vi "UHR-Fleezers Control (host) - Lorentz v3.vi"() -> ()   [LabVIEW 2014] (continued)
            n2949 = call "Volt to I16.vi"("Voltage In"=w5137) -> ("I16 Voltage Out"=w5147:i16)
            n2950 = xnode "Read/Write Control"("FPGA VI Reference In"=w5153, "error in"=w5152, "AI to FIFO"=w5149, "APD to FIFO"=w5149, "Start scan (MCL)"=w5149, "AO1"=w5148, "AO2"=w5147) -> ("FPGA VI Reference Out"=w5151:T36, "error out"=w5150:errorcluster)
          }
        }
        "Initial Y" <- w5118
        "Initial X" <- w5117
        "wait to reset values" <- w5119
      }
    }
    n2951 = xnode "Read/Write Control"("FPGA VI Reference In"=w4264) -> ("FPGA VI Reference Out"=w4223:T36, "BD1 Frequency Out 1"=w4266:u64)  [unwired: 1 in, 1 out]
    n2952 = And(x="Save scans", y=w4525) -> (x .and. y?=w4545:bool)
    n2953 = call "IR AOM word to freq.vi"("Frequency Word In (U64)"=w4266) -> ("Frequency Out (MHz)"=w4265:dbl)
    n2954 = local read "BD 1 Frequency 2 (MHz)"() -> (w4325:dbl)
    n2955 = Subtract(x=w4325, y=w4265) -> (x-y=w4318:dbl)
    "Current deltaF (MHz)" <- w4318
    n2956 = control-ref of="Piezo trap cursor control"() -> (w4224:refnum<vi>)
    n2957 = Unbundle By Name("Cursor control") -> ("X"=w4226:bool, "Y"=w4225:bool)
    n2958 = local read "APD Elements/DMA read"() -> (w4382:u32)
    n2959 = local read "Trap AI Elements/DMA read"() -> (w4512:u32)
    n2960 = case shown="False" w4226 {
      tunnel: w4224 -> [w4598 w4608]
      tunnel: w4223 -> [_ w4600]
      frame False {
        n2961 = local read "T3 X (V)"() -> (w4599:dbl)
        n2962 = property class="XYGraph (strict)"(reference=w4598, "Cursor.Cursor X"=w4599) -> ()  [unwired: 1 in, 2 out]
      }
      frame True {
        n2963 = property class="XYGraph (strict)"(reference=w4608) -> ("Cursor.Cursor X"=w4605:dbl)  [unwired: 1 in, 2 out]
        n2964 = In Range and Coerce(upper limit=10.0, x=w4605, lower limit=0.0) -> (coerced(x)=w4603:dbl)  [unwired: 1 out]
        n2965 = Multiply(x=3276.7, y=w4603) -> (x*y=w4602:dbl)
        n2966 = To Unsigned Word Integer(number=w4602) -> (unsigned 16bit integer=w4601:u16)
        n2967 = xnode "Read/Write Control"("FPGA VI Reference In"=w4600, "Piezo Trap X (AO5)"=w4601) -> ()  [unwired: 1 in, 2 out]
      }
    }
    n2968 = case shown="False" w4225 {
      tunnel: w4224 -> [w4585 w4597]
      tunnel: w4223 -> [_ w4588]
      frame False {
        n2969 = local read "T3 Y (V)"() -> (w4587:dbl)
        n2970 = Negate(x=w4587) -> (-x=w4586:dbl)
        n2971 = property class="XYGraph (strict)"(reference=w4585, "Cursor.Cursor Y"=w4586) -> ()  [unwired: 1 in, 2 out]
      }
      frame True {
        n2972 = property class="XYGraph (strict)"(reference=w4597) -> ("Cursor.Cursor Y"=w4594:dbl)  [unwired: 1 in, 2 out]
        n2973 = In Range and Coerce(upper limit=0.0, x=w4594, lower limit=-10.0) -> (coerced(x)=w4593:dbl)  [unwired: 1 out]
        n2974 = Negate(x=w4593) -> (-x=w4591:dbl)
        n2975 = Multiply(x=3276.7, y=w4591) -> (x*y=w4590:dbl)
        n2976 = To Unsigned Word Integer(number=w4590) -> (unsigned 16bit integer=w4589:u16)
        n2977 = xnode "Read/Write Control"("FPGA VI Reference In"=w4588, "Piezo Trap Y (AO4)"=w4589) -> ()  [unwired: 1 in, 2 out]
      }
    }
    n2978 = local read "Trap Pos Elements/DMA read"() -> (w4473:u32)
    n2979 = local read "DMA Update Period (s)"() -> (w4300:dbl)
    n2980 = xnode "Invoke Method"("FPGA VI Reference In"=w4477, "error in"=w4476, "Number of Elements"=w4473, "Timeout (ms)"=-1) -> ("Data"=w4445:void[], "Elements Remaining"=→"Trap Pos FIFO El Remaining")  [unwired: 2 out]
    n2981 = xnode "Get Trap Data"("FPGA VI Reference In"=w4477, "error in"=w4476, "Number of Elements"=w4512, "Timeout (ms)"=-1 ("Timeout")) -> ("FPGA VI Reference Out"=w4324:T36, "error out"=w4415:errorcluster, "Data"=w4307:void[], "Elements Remaining"=w4579)
    "FIFO El. Rem." <- w4579
    n2982 = local read "Trap AI FIFO Depth"() -> (w4581:u32)
    n2983 = xnode "Get APD Data"("FPGA VI Reference In"=w4477, "error in"=w4476, "Number of Elements"=w4382, "Timeout (ms)"=-1) -> ("Data"=w4279:void[], "Elements Remaining"=→"APD FIFO Elements Remaining")  [unwired: 2 out]
    n2984 = feedback #1(0.0) -> (w4468:dbl)
    n2985 = To Time Stamp(1:w4468) -> (0:w4262:timestamp)
    n2986 = Add(x=w4300, y=w4468) -> (x+y=w4556:dbl)
    n2987 = feedback-in #1(w4556) -> ()
    n2988 = Subtract(x=w4581, y=w4512) -> (x-y=w4580:u32)
    n2989 = local read "APD Integration Time (s)"() -> (w4271:dbl)
    n2990 = Divide(x=w4579, y=w4580) -> (x/y=w4578:dbl)
    "Buffer Status" <- w4578
    n2991 = local read "Trap Sets"() -> (w4308:u32)
    n2992 = Divide(x=w4300, y="PSD Data Period (s)") -> (x/y=w4299:dbl)
    n2993 = Equal?(x=w4578, y=1.0) -> (x = y?=w4576:bool)
    n2994 = local read "Number of APDs"() -> (w4278:u8)
    n2995 = Decimate 1D Array(w4445) -> (w4442:void[], w4444:void[], w4443:void[], w4269:void[], w4267:void[])
    n2996 = To Unsigned Long Integer(number=w4299) -> (unsigned 32bit integer=w4298:u32)
    n2997 = case "Alert buffer overflow" shown="True" w4576 {
      frame False {
      }
      frame True {
        n2998 = call <vilib>:"Beep.vi"() -> ()  [unwired: 3 in, 9 out]
        "Overflow (data lost)" <- TRUE ("Overflow (data lost)")
      }
    }
    n2999 = To Unsigned Long Integer(number=w4442) -> (unsigned 32bit integer=w4441:u32[])
    n3000 = Join Numbers(hi=w4444, lo=w4443) -> ((hi.lo)=w4440:u32)
    n3001 = Divide(x=w4269, y=w4268) -> (x/y=w4250:dbl)
    n3002 = Divide(x=w4267, y=w4268) -> (x/y=w4249:dbl)
    n3003 = call "Arduino input-output.vi"("VISA resource name"=w4303, "Sets to read"=w4298, "Error in"=w4302) -> ("VISA resource out"=w4297:refnum<visa-resource-name>, "Channel names"=w4287:string[], "Output"=w4286:dbl[][], "Error out"=→"Serial Error out":errorcluster)
    n3004 = call "deinterlace.vi"("Detector type"="Detector Type", "Data"=w4307, "Trap sets"=w4308, "Flip x sign"="Flip X Sign") -> ("Channel pattern"=w4304:i32, "Channel names"=w4283:string[], "Deinterlaced normalized data"=w4284:dbl[][], "Deinterlaced data"=w4305:i16[])
    n3005 = Join Numbers(hi=w4441, lo=w4440) -> ((hi.lo)=w4435:u64[])
    n3006 = local read "Data Period (s)"() -> (w4256:dbl)
    n3007 = call "APD data extraction.vi"("Data"=w4279, "Number of APD's"=w4278, "APD integration time (s)"=w4271, "APD Ave N"="APD Ave N", "APD Disp. Downsample"="APD Disp. Downsample", "APD Disp. Scale"="APD Disp. Scale", "Time Stamp"=w4262) -> ("Output cluster"=→"APD rates cluster":T1, "Output Data"=w4274:T60, "Output waveform"=w4273:waveform(dbl)[], "APD Display period (s)"=w4272:dbl)
    "APD Display Period (s)" <- w4272
    n3008 = call "IR AOM word to freq - vec.vi"("Frequency Word In (double vec)"=w4435) -> ("Frequency Out"=w4472:dbl[])
    n3009 = Decimate 1D Array(w4249) -> (w4246:dbl[], w4245:dbl[])
    n3010 = Decimate 1D Array(w4250) -> (w4248:dbl[], w4247:dbl[])
    n3011 = Add(x=w4248, y=w4247) -> (x+y=w4244:dbl[])
    n3012 = Add(x=w4246, y=w4245) -> (x+y=w4243:dbl[])
    n3013 = Decimate 1D Array(w4472) -> (w4471:dbl[], w4470:dbl[])
    n3014 = Divide(x=w4244, y=w4242) -> (x/y=w4240:dbl[])
    n3015 = Divide(x=w4243, y=w4242) -> (x/y=w4241:dbl[])
    n3016 = Reciprocal(x=w4272) -> (1/x=→"APD Display Freq. (Hz)":dbl)
    n3017 = call "Generate Waveform.vi"("Downsampling"="PSD downsample", "Data Period (s)"="PSD Data Period (s)", "Data"=w4286, "Plot names"=w4287, "Time Stamp"=w4262) -> ("Downsampled data"=w4285:waveform(dbl)[])  [unwired: 1 out]
    n3018 = Build Array(w4471, w4470, w4240, w4241) -> (w4263:dbl[][])
    n3019 = for {
      tunnel: w4286 -> [w4624] mode=indexing
      tunnel: [w4623] -> w4293 mode=indexing
      n3020 = call-poly <vilib>:"Mean.vi"("X"=w4624) -> ("mean"=w4623:dbl)  [unwired: 1 out]
    }
    n3021 = Multiply(x=w4256, y="Trap Disp. Downsample") -> (x*y=w4469:dbl)
    "Display Period (s)" <- w4469
    n3022 = for {
      tunnel: w4284 -> [w4626] mode=indexing
      tunnel: [w4625] -> w4292 mode=indexing
      n3023 = call-poly <vilib>:"Mean.vi"("X"=w4626) -> ("mean"=w4625:dbl)  [unwired: 1 out]
    }
    n3024 = call "Generate Waveform.vi"("Downsampling"="Trap Disp. Downsample", "Data Period (s)"=w4256, "Data"=w4284, "Plot names"=w4283, "Time Stamp"=w4262) -> ("Downsampled data"=w4281:waveform(dbl)[], "Non downsampled waveform"=w4280:waveform(dbl)[])
    n3025 = Multiply(x="APD Disp. Scale", y=w4273) -> (x*y=w4490:waveform(dbl)[])
    n3026 = Reciprocal(x=w4469) -> (1/x=→"Trap Disp. Freq. (Hz)":dbl)
    n3027 = Insert Into Array(array=w4293, index=0, new element=w4292) -> (→"Values":dbl[])
    n3028 = Multiply(x="APD Disp. Downsample", y=w4271) -> (x*y=w4489:dbl)
    n3029 = Decimate 1D Array(w4305) -> (w4460:i16[], w4459:i16[], w4457:i16[], w4456:i16[])  [unwired: 9 out]
    n3030 = Divide(x=w4490, y=w4489) -> (x/y=w4387:waveform(dbl)[])
    n3031 = Insert Into Array(array=w4287, index=0, new element=w4283) -> (→"AI labels":string[])
    n3032 = case shown="1" "Plot Trap Positions" {
      tunnel: [w4609 w4618] -> w4257
      frame 0, Default {
        n3033 = local read "BD 1 Frequency 2 (MHz)"() -> (w4612:dbl)
        n3034 = local read "BD 1 Frequency 1 (MHz)"() -> (w4613:dbl)
        n3035 = local read "T3 Y (V)"() -> (w4610:dbl)
        n3036 = local read "T3 X (V)"() -> (w4611:dbl)
        n3037 = Build Array(w4613, w4612, w4611, w4610) -> (w4609:dbl[])
      }
      frame 1 {
        w4617 = 75.0
        n3038 = Unbundle By Name("Piezo trap 0 position relative to 75 MHz") -> ("X (V)"=w4615:dbl, "Y (V)"=w4614:dbl)
        n3039 = Build Array(w4617, w4617, w4615, w4614) -> (w4618:dbl[])
      }
    }
    n3040 = Divide(x=w4460, y=w4459) -> (x/y=w4461:dbl[])
    n3041 = Divide(x=w4457, y=w4456) -> (x/y=w4458:dbl[])
    n3042 = local read "AOM X Cal (nm/MHz)"() -> (w4259:dbl)
    n3043 = Split 1D Array(array=w4461, index="N El. to Ave.") -> (second subarray=w4464:dbl[])  [unwired: 1 out]
    n3044 = Split 1D Array(array=w4458, index="N El. to Ave.") -> (second subarray=w4463:dbl[])  [unwired: 1 out]
    n3045 = Index Array(array=w4387, index=0) -> (element=w4485:waveform(dbl))
    n3046 = Index Array(array=w4387, index=1) -> (element=w4483:waveform(dbl))
    n3047 = Index Array(array=w4387, index=2) -> (element=w4389:waveform(dbl))
    n3048 = call-poly <vilib>:"Mean.vi"("X"=w4464) -> ("mean"=w4452:dbl)  [unwired: 1 out]
    n3049 = call-poly <vilib>:"Mean.vi"("X"=w4463) -> ("mean"=w4451:dbl)  [unwired: 1 out]
    n3050 = Subtract(x=w4485, y="APD 1 Offset") -> (x-y=w4481:waveform(dbl))
    n3051 = Subtract(x=w4483, y="APD 2 Offset") -> (x-y=w4480:waveform(dbl))
    n3052 = Subtract(x=w4389, y="APD 3 Offset") -> (x-y=w4386:waveform(dbl))
    n3053 = Build Array(w4481, w4480, w4386) -> (→"APD Chart":waveform(dbl)[])
    n3054 = Build Array(w4259, w4259, "Piezo Trap X cal (nm/V)", "Piezo Trap Y cal (nm/V)") -> (w4258:dbl[])
    n3055 = local read "Trap X AI1 (DMA)"() -> (w4462:T19)
    n3056 = To Fixed-Point(number=w4451) -> (fixed-point=w4449:fxp<+/-,16,1>)  [unwired: 1 in]
    n3057 = To Fixed-Point(number=w4452) -> (fixed-point=w4450:fxp<+/-,16,1>)  [unwired: 1 in]
    n3058 = Cluster To Array(cluster="Negate Axis") -> (array=w4251:bool[])
    n3059 = call "Generate Trap Positiion Waveform.vi"("Base trap positions"=w4257, "Data Period (s)"=w4256, "Input data"=w4263, "Position calibration values"=w4258, "Trap Pos. Disp. Downsample (s)"="Trap Pos. Disp. Downsample", "Negate axis"=w4251, "Time Stamp"=w4262) -> ("Output waveforms"=w4228:waveform(dbl)[])  [unwired: 3 in]
    "Trap Positions" <- w4228
    n3060 = Bundle By Name(cluster=w4462, "Set 1"=w4450, "Set 2"=w4449) -> (→"Trap X AI1 (DMA)":T19)
    n3061 = Initialize Array(0.0) -> (w4253:dbl[][])  [unwired: 2 in]
    n3062 = local read "Display Period (s)"() -> (w4499:dbl)
    n3063 = for {
      tunnel: w4228 -> [w4622] mode=indexing
      shift-right: [w4620] -> w4230
      shift-left: w4253 -> [w4621]
      n3064 = Unbundle By Name(w4622) -> ("Y"=w4619:dbl[])
      n3065 = Build Array (concatenate)(w4621, w4619) -> (w4620:dbl[][])
    }
    n3066 = Build Array (concatenate)(w4273, w4281, w4285) -> (w4294:waveform(dbl)[])
    "All Signals" <- w4294
    n3067 = Divide(x="Bead Sep. Int. Time (s)", y=w4499) -> (x/y=w4236:dbl)
    n3068 = feedback #2(w4230) -> (w4237:dbl[][])
    n3069 = call "Trap Pos RMS.vi"("Accumulated array"=w4237, "New Array"=w4230, "Number of sets to average"=w4236) -> ("Output accumulated array"=w4235:dbl[][], "RMS"=w4233:dbl[], "Mean"=w4234:dbl[])
    n3070 = feedback-in #2(w4235) -> ()
    n3071 = Index Array(array=w4230, index (row)=0 ("index")) -> (element=w4229:dbl[])  [unwired: 1 in]
    n3072 = Array To Cluster(array=w4233) -> (cluster=→"Trap RMS (ang)":T61)
    n3073 = Array To Cluster(array=w4234) -> (cluster=→"Mean Trap Positions (nm)":T62)
    n3074 = local read "Data points/scans (MCL)"() -> (w4539:dbl)
    n3075 = Unbundle(w4274) -> ("APD 1"=w4385:u32[])  [unwired: 2 out]
    n3076 = To Double Precision Float(number=w4385) -> (double precision float=w4507:dbl[])
    n3077 = Increment(x=w4539) -> (x+1=w4540:dbl)
    n3078 = feedback #3(w4540) -> (w4543:dbl)
    n3079 = Select(t=0, s=w4530, f=w4543) -> (s? t:f=w4536:dbl)
    n3080 = Array Size(array=w4507) -> (size(s)=w4542:i32)
    n3081 = Add(x=w4542, y=w4536) -> (x+y=w4537:dbl)
    n3082 = Greater?(x=w4537, y=w4539) -> (0:w4538:bool)
    n3083 = Select(t=w4536, s=w4538, f=w4537) -> (s? t:f=w4535:dbl)
    n3084 = feedback-in #3(w4535) -> ()
    n3085 = local read "MCL Scanning"() -> (w4533:bool)
    n3086 = Index Array(array=w4281, index="index 1") -> (element=w4377:waveform(dbl))
    n3087 = Index Array(array=w4281, index="index 2") -> (element=w4381:waveform(dbl))
    n3088 = Unbundle By Name(w4377) -> ("Y"=w4376:dbl[])
    n3089 = Unbundle By Name(w4381) -> ("Y"=w4380:dbl[])
    n3090 = Not(x=w4538) -> (.not. x?=w4532:bool)
    n3091 = And(x=w4532, y=w4533) -> (x .and. y?=w4534:bool)
    n3092 = call-poly <vilib>:"Mean.vi"("X"=w4376) -> ("mean"=→"Trap 1 sum mean":dbl)  [unwired: 1 out]
    n3093 = call-poly <vilib>:"Mean.vi"("X"=w4380) -> ("mean"=→"Trap 2 sum mean":dbl)  [unwired: 1 out]
    n3094 = Or(x=w4534, y=w4530) -> (x .or. y?=w4531:bool)
    n3095 = Equal?(x="Tab Control 6", y=T52."High Res Display") -> (x = y?=w4509:bool)
    n3096 = case shown="True" "X or Y?" {
      tunnel: w4281 -> [w4735 w4741]
      tunnel: [w4736 w4740] -> w4351
      tunnel: [w4734 w4739] -> w4348
      frame False {
        n3097 = Index Array(array=w4735, index=0) -> (element=w4736:waveform(dbl))
        n3098 = Index Array(array=w4735, index=3) -> (element=w4734:waveform(dbl))
      }
      frame True {
        n3099 = Index Array(array=w4741, index=1) -> (element=w4740:waveform(dbl))
        n3100 = Index Array(array=w4741, index=4) -> (element=w4739:waveform(dbl))
      }
    }
    n3101 = case "For displaying the high resolution display (no downsampling)" shown="True" w4509 {
      tunnel: w4280 -> [_ w4874]
      frame False {
      }
      frame True {
        n3102 = Index Array(array=w4874, index="High Res. Display") -> (element=w4875:waveform(dbl))
        n3103 = call <vilib>:"Std Deviation and Variance.vi"("X"=w4875) -> ("mean"=w4882:dbl, "standard deviation"=w4887:dbl)  [unwired: 1 in, 1 out]
        "Mean Intensity" <- w4882
        "Sigma" <- w4887
        n3104 = Subtract(x=w4875, y=w4882) -> (x-y=w4881:waveform(dbl))
        n3105 = Select(t=w4881, s="Subtract mean", f=w4875) -> (s? t:f=→"1 Channel":waveform(dbl))
        n3106 = Divide(x=w4887, y=w4882) -> (x/y=→"Sigma/Mean":dbl)
        n3107 = feedback #4(1) -> (w4876:i32)
        n3108 = Greater Or Equal?(x=w4876, y="Slow mean N ave.") -> (x >= y?=w4889:bool)
        n3109 = Increment(x=w4876) -> (x+1=w4891:i32)
        n3110 = Select(t=1, s=w4889, f=w4891) -> (s? t:f=w4878:i32)
        n3111 = feedback-in #4(w4878) -> ()
        n3112 = feedback #5() -> (w4879:waveform(dbl))  [unwired: 1 out]
        n3113 = case shown="Default" w4876 {
          tunnel: [w4894 w4897] -> w4880
          tunnel: w4879 -> [w4896 _]
          tunnel: w4875 -> [w4895 w4897]
          frame Default {
            n3114 = call-poly <vilib>:"Append Waveforms.vi"("waveform B"=w4895, "waveform A"=w4896) -> ("waveform out"=w4894:waveform(dbl))  [unwired: 1 in, 8 out]
          }
          frame 1 {
          }
        }
        n3115 = feedback-in #5(w4880) -> ()
        n3116 = case shown="True" w4889 {
          tunnel: w4880 -> [_ w4893]
          frame False {
          }
          frame True {
            n3117 = call-poly <vilib>:"Mean.vi"("X"=w4893) -> ("mean"=→"Slow mean":dbl)  [unwired: 1 out]
          }
        }
      }
    }
    n3118 = case "For plotting results of scanning MCL (fluorescence and detection laser images)" shown="True" w4531 {
      tunnel: w4530 -> [_ w4975]
      tunnel: w4539 -> [_ _]
      tunnel: w4280 -> [_ w5071]
      tunnel: w4478 -> [_ w5003]
      tunnel: w4274 -> [_ w4981]
      frame False {
      }
      frame True {
        w4941 = u32 0 items=["Horizontal", "Vertical", "Central", "1st Diagonal", "2nd Diagonal"] ("Type of Symmetry")
        w4948 = u32 0 items=["Horizontal", "Vertical", "Central", "1st Diagonal", "2nd Diagonal"] ("Type of Symmetry")
        w4955 = u32 0 items=["Horizontal", "Vertical", "Central", "1st Diagonal", "2nd Diagonal"] ("Type of Symmetry")
        w4958 = u32 0 items=["Horizontal", "Vertical", "Central", "1st Diagonal", "2nd Diagonal"] ("Type of Symmetry")
        w4965 = u32 0 items=["Horizontal", "Vertical", "Central", "1st Diagonal", "2nd Diagonal"] ("Type of Symmetry")
        n3119 = Unbundle(w4981) -> ("APD 1"=w4980:u32[], "APD 2"=w4978:u32[], "APD 3"=w4976:u32[])
        n3120 = To Double Precision Float(number=w4980) -> (double precision float=w4979:dbl[])
        n3121 = To Double Precision Float(number=w4978) -> (double precision float=w4977:dbl[])
        n3122 = To Double Precision Float(number=w4976) -> (double precision float=w4969:dbl[])
        n3123 = Index Array(array=w5071, index=10) -> (element=w5077:waveform(dbl))
        n3124 = Index Array(array=w5071, index=11) -> (element=w5074:waveform(dbl))
        n3125 = local read "Cycles/step (MCL)"() -> (w5033:u64)
        n3126 = Index Array(array=w5071, index="Channel") -> (element=w5073:waveform(dbl))
        n3127 = Unbundle(w5003) -> ("New Image"=w5002:T6, "New Image"=w5001:T6, "New Image"=w4982:T6, "New Image"=w4983:T6, "New Image"=w4984:T6)
        n3128 = local read "Scan steps (MCL)"() -> (w4971:u64)
        n3129 = Unbundle By Name(w5077) -> ("Y"=w5035:dbl[])
        n3130 = Unbundle By Name(w5074) -> ("Y"=w5037:dbl[])
        n3131 = local read "Scan lines (y)"() -> (w4972:u64)
        n3132 = local read "N APD Samp/step"() -> (w4974:dbl)
        n3133 = Unbundle By Name(w5073) -> ("Y"=w5042:dbl[])
        n3134 = call "downsample 1D array - double.vi"("Ave N"=w5033, "Array In"=w5035) -> ("Array Out"=w5034:dbl[])  [unwired: 1 out]
        n3135 = call "downsample 1D array - double.vi"("Ave N"=w5033, "Array In"=w5037) -> ("Array Out"=w5036:dbl[])  [unwired: 1 out]
        n3136 = call "downsample 1D array - double.vi"("Ave N"=w5033, "Array In"=w5042) -> ("Array Out"=w5041:dbl[])  [unwired: 1 out]
        n3137 = Multiply(x=w4971, y=u64 2) -> (x*y=w4973:u64)
        n3138 = feedback #6(w4977) -> (w5021:dbl[])
        n3139 = Build Array (concatenate)(w5021, w4977) -> (w5020:dbl[])
        n3140 = feedback #7(w4969) -> (w4970:dbl[])
        n3141 = Build Array (concatenate)(w4970, w4969) -> (w4968:dbl[])
        n3142 = Select(t=w4977, s=w4975, f=w5020) -> (s? t:f=w5005:dbl[])
        n3143 = feedback-in #6(w5005) -> ()
        n3144 = Select(t=w4969, s=w4975, f=w4968) -> (s? t:f=w4986:dbl[])
        n3145 = feedback-in #7(w4986) -> ()
        n3146 = feedback #8(w4979) -> (w5096:dbl[])
        n3147 = Build Array (concatenate)(w5096, w4979) -> (w5079:dbl[])
        n3148 = Select(t=w4979, s=w4975, f=w5079) -> (s? t:f=w5083:dbl[])
        n3149 = feedback-in #8(w5083) -> ()
        n3150 = feedback #9(w5034) -> (w5085:dbl[])
        n3151 = Build Array (concatenate)(w5085, w5034) -> (w5076:dbl[])
        n3152 = feedback #10(w5041) -> (w5094:dbl[])
        n3153 = Build Array (concatenate)(w5094, w5041) -> (w5093:dbl[])
        n3154 = feedback #11(w5036) -> (w5087:dbl[])
        n3155 = Build Array (concatenate)(w5087, w5036) -> (w5088:dbl[])
        n3156 = Select(t=w5034, s=w4975, f=w5076) -> (s? t:f=w5038:dbl[])
        n3157 = feedback-in #9(w5038) -> ()
        n3158 = Select(t=w5041, s=w4975, f=w5093) -> (s? t:f=w5040:dbl[])
        n3159 = feedback-in #10(w5040) -> ()
        n3160 = Select(t=w5036, s=w4975, f=w5088) -> (s? t:f=w5039:dbl[])
        n3161 = feedback-in #11(w5039) -> ()
        n3162 = call "integrate 1D array interval - double.vi"("Ave N"=w4974, "Array In"=w5005) -> ("Array Out"=w5016:dbl[])  [unwired: 1 out]
        n3163 = call "integrate 1D array interval - double.vi"("Ave N"=w4974, "Array In"=w4986) -> ("Array Out"=w4997:dbl[])  [unwired: 1 out]
        n3164 = call "integrate 1D array interval - double.vi"("Ave N"=w4974, "Array In"=w5083) -> ("Array Out"=w5082:dbl[])  [unwired: 1 out]
        n3165 = Array Size(array=w5016) -> (size(s)=w5017:i32)
        n3166 = Array Size(array=w4997) -> (size(s)=w4998:i32)
        n3167 = Array Size(array=w5082) -> (size(s)=w5084:i32)
        n3168 = Multiply(x=w4972, y=w4973) -> (x*y=w5019:u64)
        n3169 = Multiply(x=w4972, y=w4973) -> (x*y=w5000:u64)
        n3170 = Multiply(x=w4972, y=w4973) -> (x*y=w5092:u64)
        n3171 = Subtract(x=w5019, y=w5017) -> (x-y=w5010:u64)
        n3172 = call-poly <vilib>:"Mean.vi"("X"=w5016) -> ("mean"=w5007:dbl)  [unwired: 1 out]
        n3173 = Subtract(x=w5000, y=w4998) -> (x-y=w4991:u64)
        n3174 = call-poly <vilib>:"Mean.vi"("X"=w4997) -> ("mean"=w4988:dbl)  [unwired: 1 out]
        n3175 = Subtract(x=w5092, y=w5084) -> (x-y=w5032:u64)
        n3176 = call-poly <vilib>:"Mean.vi"("X"=w5082) -> ("mean"=w5029:dbl)  [unwired: 1 out]
        n3177 = call-poly <vilib>:"Mean.vi"("X"=w5038) -> ("mean"=w5022:dbl)  [unwired: 1 out]
        n3178 = call-poly <vilib>:"Mean.vi"("X"=w5040) -> ("mean"=w5027:dbl)  [unwired: 1 out]
        n3179 = call-poly <vilib>:"Mean.vi"("X"=w5039) -> ("mean"=w5025:dbl)  [unwired: 1 out]
        n3180 = Initialize Array(1.0 ("element"), w5010) -> (w5006:dbl[])
        n3181 = Initialize Array(1.0 ("element"), w4991) -> (w4987:dbl[])
        n3182 = Initialize Array(1.0 ("element"), w5032) -> (w5023:dbl[])
        n3183 = Multiply(x=w5006, y=w5007) -> (x*y=w5008:dbl[])
        n3184 = Multiply(x=w4987, y=w4988) -> (x*y=w4989:dbl[])
        n3185 = Multiply(x=w5023, y=w5029) -> (x*y=w5030:dbl[])
        n3186 = Multiply(x=w5023, y=w5025) -> (x*y=w5026:dbl[])
        n3187 = Multiply(x=w5023, y=w5027) -> (x*y=w5028:dbl[])
        n3188 = Multiply(x=w5023, y=w5022) -> (x*y=w5024:dbl[])
        n3189 = Build Array (concatenate)(w5016, w5008) -> (w5018:dbl[])
        n3190 = Build Array (concatenate)(w4997, w4989) -> (w4999:dbl[])
        n3191 = Build Array (concatenate)(w5082, w5030) -> (w5091:dbl[])
        n3192 = Build Array (concatenate)(w5038, w5024) -> (w5086:dbl[])
        n3193 = Build Array (concatenate)(w5040, w5028) -> (w5090:dbl[])
        n3194 = Build Array (concatenate)(w5039, w5026) -> (w5089:dbl[])
        n3195 = Reshape Array(w5018, w4972, w4973) -> (w5014:dbl[][])
        n3196 = Reshape Array(w4999, w4972, w4973) -> (w4995:dbl[][])
        n3197 = Reshape Array(w5091, w4972, w4973) -> (w5069:dbl[][])
        n3198 = Reshape Array(w5086, w4972, w4973) -> (w5052:dbl[][])
        n3199 = Reshape Array(w5090, w4972, w4973) -> (w5044:dbl[][])
        n3200 = Reshape Array(w5089, w4972, w4973) -> (w5059:dbl[][])
        n3201 = Array Subset(array=w5014, index (col)=0 ("index"), length (col)=w4971) -> (w5013:dbl[][])  [unwired: 2 in]
        n3202 = Array Subset(array=w5014, index (col)=w4971) -> (w5011:dbl[][])  [unwired: 3 in]
        n3203 = Array Subset(array=w4995, index (col)=0 ("index"), length (col)=w4971) -> (w4994:dbl[][])  [unwired: 2 in]
        n3204 = Array Subset(array=w4995, index (col)=w4971) -> (w4992:dbl[][])  [unwired: 3 in]
        n3205 = Array Subset(array=w5059, index (col)=0 ("index"), length (col)=w4971) -> (w5064:dbl[][])  [unwired: 2 in]
        n3206 = Array Subset(array=w5059, index (col)=w4971) -> (w5062:dbl[][])  [unwired: 3 in]
        n3207 = Array Subset(array=w5069, index (col)=0 ("index"), length (col)=w4971) -> (w5068:dbl[][])  [unwired: 2 in]
        n3208 = Array Subset(array=w5069, index (col)=w4971) -> (w5066:dbl[][])  [unwired: 3 in]
        n3209 = Array Subset(array=w5044, index (col)=0 ("index"), length (col)=w4971) -> (w5050:dbl[][])  [unwired: 2 in]
        n3210 = Array Subset(array=w5044, index (col)=w4971) -> (w5048:dbl[][])  [unwired: 3 in]
        n3211 = Array Subset(array=w5052, index (col)=0 ("index"), length (col)=w4971) -> (w5057:dbl[][])  [unwired: 2 in]
        n3212 = Array Subset(array=w5052, index (col)=w4971) -> (w5055:dbl[][])  [unwired: 3 in]
        n3213 = for {
          tunnel: w5013 -> [w5100] mode=indexing
          tunnel: [w5099] -> w5012 mode=indexing
          workers-P: _ -> [_]
          n3214 = Reverse 1D Array(array=w5100) -> (reversed array=w5099:dbl[])
        }
        n3215 = for {
          tunnel: w4994 -> [w5098] mode=indexing
          tunnel: [w5097] -> w4993 mode=indexing
          workers-P: _ -> [_]
          n3216 = Reverse 1D Array(array=w5098) -> (reversed array=w5097:dbl[])
        }
        n3217 = for {
          tunnel: w5064 -> [w5106] mode=indexing
          tunnel: [w5105] -> w5063 mode=indexing
          workers-P: _ -> [_]
          n3218 = Reverse 1D Array(array=w5106) -> (reversed array=w5105:dbl[])
        }
        n3219 = for {
          tunnel: w5068 -> [w5108] mode=indexing
          tunnel: [w5107] -> w5067 mode=indexing
          workers-P: _ -> [_]
          n3220 = Reverse 1D Array(array=w5108) -> (reversed array=w5107:dbl[])
        }
        n3221 = for {
          tunnel: w5050 -> [w5102] mode=indexing
          tunnel: [w5101] -> w5049 mode=indexing
          workers-P: _ -> [_]
          n3222 = Reverse 1D Array(array=w5102) -> (reversed array=w5101:dbl[])
        }
        n3223 = for {
          tunnel: w5057 -> [w5104] mode=indexing
          tunnel: [w5103] -> w5056 mode=indexing
          workers-P: _ -> [_]
          n3224 = Reverse 1D Array(array=w5104) -> (reversed array=w5103:dbl[])
        }
        n3225 = Index Array(array=w5069, index (row)=0) -> (element=→"Waveform Graph":dbl[])  [unwired: 1 in]
        n3226 = Add(x=w5012, y=w5011) -> (x+y=w5004:dbl[][])
        n3227 = Add(x=w4993, y=w4992) -> (x+y=w4985:dbl[][])
        n3228 = Add(x=w5063, y=w5062) -> (x+y=w5061:dbl[][])
        n3229 = Add(x=w5067, y=w5066) -> (x+y=w5043:dbl[][])
        n3230 = Add(x=w5049, y=w5048) -> (x+y=w5047:dbl[][])
        n3231 = Add(x=w5056, y=w5055) -> (x+y=w5054:dbl[][])
        n3232 = Divide(x=w5047, y=2) -> (x/y=w5045:dbl[][])
        n3233 = Divide(x=w5061, y=2) -> (x/y=w4951:dbl[][])
        n3234 = To Single Precision Float(number=w5043) -> (single precision float=w4964:sgl[][])
        n3235 = To Single Precision Float(number=w5004) -> (single precision float=w4947:sgl[][])
        n3236 = To Single Precision Float(number=w4985) -> (single precision float=w4940:sgl[][])
        n3237 = Divide(x=w5054, y=2) -> (x/y=w4953:dbl[][])
        n3238 = Transpose 2D Array(2D array=w5045) -> (transposed array=→"Data map":dbl[][])
        n3239 = To Single Precision Float(number=w4951) -> (single precision float=w4957:sgl[][])
        n3240 = To Single Precision Float(number=w4953) -> (single precision float=w4954:sgl[][])
        n3241 = call "IMAQ ArrayToImage"("Image Pixels (Float)"=w4964, "Image"=w5002) -> ("Image Out"=w4966:T6)  [unwired: 8 in, 1 out]
        n3242 = call "IMAQ ArrayToImage"("Image Pixels (Float)"=w4947, "Image"=w5001) -> ("Image Out"=w4949:T6)  [unwired: 8 in, 1 out]
        n3243 = call "IMAQ ArrayToImage"("Image Pixels (Float)"=w4940, "Image"=w4982) -> ("Image Out"=w4942:T6)  [unwired: 8 in, 1 out]
        n3244 = call "IMAQ ArrayToImage"("Image Pixels (Float)"=w4957, "Image"=w4983) -> ("Image Out"=w4959:T6)  [unwired: 8 in, 1 out]
        n3245 = call "IMAQ Symmetry"("Type of Symmetry"=w4965, "Image Src"=w4966) -> ("Image Dst Out"=w4962:T6)  [unwired: 3 in, 1 out]
        n3246 = call "IMAQ ArrayToImage"("Image Pixels (Float)"=w4954, "Image"=w4984) -> ("Image Out"=w4956:T6)  [unwired: 8 in, 1 out]
        n3247 = call "IMAQ Symmetry"("Type of Symmetry"=w4948, "Image Src"=w4949) -> ("Image Dst Out"=w4945:T6)  [unwired: 3 in, 1 out]
        n3248 = call "IMAQ Symmetry"("Type of Symmetry"=w4941, "Image Src"=w4942) -> ("Image Dst Out"=w4938:T6)  [unwired: 3 in, 1 out]
        n3249 = call "IMAQ Symmetry"("Type of Symmetry"=w4958, "Image Src"=w4959) -> ("Image Dst Out"=→"Detection Laser X":T6)  [unwired: 3 in, 1 out]
        n3250 = call "IMAQ Symmetry"("Type of Symmetry"=w4955, "Image Src"=w4956) -> ("Image Dst Out"=→"Detection Laser Y":T6)  [unwired: 3 in, 1 out]
        n3251 = call "IMAQ Set Simple Calibration"("Calibration Axis Info"=T53 {"Origin Pixel"={"X"=0.0, "Y"=0.0}, "Angle Relative to Horizontal (deg)"=0.0, "Axis Reference"=0}, "Grid Descriptor"=T54 {"X Step"=0.3, "Y Step"=0.3, "Unit"=enum."Undefined"}, "Image"=w4962) -> ("Calibrated Image"=→"APD 1":T6)  [unwired: 7 in, 1 out]
        n3252 = call "IMAQ Set Simple Calibration"("Calibration Axis Info"=T53 {"Origin Pixel"={"X"=0.0, "Y"=0.0}, "Angle Relative to Horizontal (deg)"=0.0, "Axis Reference"=0}, "Grid Descriptor"=T54 {"X Step"=0.3, "Y Step"=0.3, "Unit"=enum."Undefined"}, "Image"=w4945) -> ("Calibrated Image"=→"APD 2":T6)  [unwired: 7 in, 1 out]
        n3253 = call "IMAQ Set Simple Calibration"("Calibration Axis Info"=T53 {"Origin Pixel"={"X"=0.0, "Y"=0.0}, "Angle Relative to Horizontal (deg)"=0.0, "Axis Reference"=0}, "Grid Descriptor"=T54 {"X Step"=0.3, "Y Step"=0.3, "Unit"=enum."Undefined"}, "Image"=w4938) -> ("Calibrated Image"=→"APD 3":T6)  [unwired: 7 in, 1 out]
      }
    }
    n3254 = case "For computing FFTs for display" shown="True" "Compute FFT" {
      tunnel: w4280 -> [_ w5255]
      frame False {
      }
      frame True {
        n3255 = Build Array("FFT 1 Choice 1", "FFT 1 Choice 2", "FFT 2 Choice 1", "FFT 2 Choice 2") -> (w5248:u16[])
        n3256 = Array Size(array=w5255) -> (size(s)=w5254:i32)
        n3257 = feedback-in #12(w5248) -> ()
        n3258 = feedback #12(u16[] [100, 100, 100, 100]) -> (w5249:u16[])
        n3259 = feedback-in #13("# Spectra to Ave.") -> ()
        n3260 = feedback #13("# Spectra to Ave.") -> (w5246:dbl)
        n3261 = Not Equal?(x="# Spectra to Ave.", y=w5246) -> (x != y?=w5245:bool)
        n3262 = Not Equal?(x=w5248, y=w5249) -> (x != y?=w5247:bool)
        n3263 = feedback #14(1.0) -> (w5232:dbl)
        n3264 = Compound Arithmetic op=OR("Reset FFT", w5247, w5245) -> (w5230:bool)
        n3265 = Select(t=1.0, s=w5230, f=w5232) -> (s? t:f=w5234:dbl)
        n3266 = Greater?(x=w5234, y="# Spectra to Ave.") -> (0:w5253:bool)
        n3267 = Increment(x=w5234) -> (x+1=w5233:dbl)
        n3268 = feedback-in #14(w5233) -> ()
        n3269 = local read "DMA Update Period (s)"() -> (w5228:dbl)
        n3270 = Multiply(x="# Spectra to Ave.", y=w5228) -> (x*y=→"Ave. Time (s)":dbl)
        n3271 = Build Array(cluster{"f0":dbl, "df":dbl, "magnitude":dbl[]} {"f0"=0.0, "df"=0.0, "magnitude"=[]} ("PSD")) -> (w5237:cluster{"f0":dbl, "df":dbl, "magnitude":dbl[]}[])
        n3272 = Build Array(w5237, w5237, w5237, w5237) -> (w5239:T63)
        n3273 = feedback #15(w5239) -> (w5244:T63)
        n3274 = for {
          N: 4 -> [_]
          tunnel: w5248 -> [w5277] mode=indexing
          tunnel: w5255 -> [w5278]
          tunnel: w5254 -> [w5280]
          tunnel: w5230 -> [w5273]
          tunnel: w5253 -> [w5272]
          tunnel: "# Spectra to Ave." -> [w5271]
          tunnel: [w5270] -> w5243 mode=indexing
          tunnel: w5244 -> [w5275] mode=indexing
          tunnel: [w5274] -> w5231 mode=indexing
          tunnel: w5234 -> [w5269]
          n3275 = Less?(x=w5277, y=w5280) -> (x < y?=w5279:bool)
          n3276 = Index Array(array=w5278, index=w5277) -> (element=w5276:waveform(dbl))
          n3277 = case shown="True" w5279 {
            tunnel: w5276 -> [_ w5297]
            tunnel: w5275 -> [w5282 w5295]
            tunnel: [w5282 w5283] -> w5274
            tunnel: w5273 -> [_ w5294]
            tunnel: w5272 -> [_ w5287]
            tunnel: w5271 -> [_ w5286]
            tunnel: [cluster{"f0":dbl, "df":dbl, "magnitude":dbl[]} {"f0"=0.0, "df"=0.0, "magnitude"=[]} ("PSD") w5288] -> w5270
            tunnel: w5269 -> [_ w5285]
            frame False {
            }
            frame True {
              n3278 = call <vilib>:"Std Deviation and Variance.vi"("X"=w5297) -> ("mean"=w5298:dbl)  [unwired: 1 in, 2 out]
              n3279 = Subtract(x=w5297, y=w5298) -> (x-y=w5296:waveform(dbl))
              n3280 = xnode "Spectral Measurements"("Signals"=w5296) -> ("PSD"=w5290:cluster{"f0":dbl, "df":dbl, "magnitude":dbl[]})  [unwired: 1 in, 1 out]
              n3281 = case shown="False" w5294 {
                tunnel: w5295 -> [w5307 _]
                tunnel: [w5303 w5312] -> w5283
                tunnel: w5290 -> [w5306 w5313]
                tunnel: w5287 -> [w5305 _]
                frame False {
                  n3282 = Build Array (concatenate)(w5307, w5306) -> (w5304:cluster{"f0":dbl, "df":dbl, "magnitude":dbl[]}[])
                  n3283 = case shown="True" w5305 {
                    tunnel: w5304 -> [w5308 w5311]
                    tunnel: [w5308 w5309] -> w5303
                    frame False {
                    }
                    frame True {
                      n3284 = Delete From Array(array=w5311, index=0) -> (array with subset deleted=w5309:cluster{"f0":dbl, "df":dbl, "magnitude":dbl[]}[])  [unwired: 1 in, 1 out]
                    }
                  }
                }
                frame True {
                  n3285 = Build Array(w5313) -> (w5312:cluster{"f0":dbl, "df":dbl, "magnitude":dbl[]}[])
                }
              }
              n3286 = for {
                tunnel: w5283 -> [w5302] mode=indexing
                tunnel: [w5301] -> w5293 mode=indexing
                workers-P: _ -> [_]
                n3287 = Unbundle By Name(w5302) -> ("magnitude"=w5301:dbl[])
              }
              n3288 = Transpose 2D Array(2D array=w5293) -> (transposed array=w5292:dbl[][])
              n3289 = for {
                tunnel: w5292 -> [w5300] mode=indexing
                tunnel: [w5299] -> w5291 mode=indexing
                workers-P: _ -> [_]
                n3290 = Add Array Elements(numeric array=w5300) -> (sum=w5299:dbl)
              }
              n3291 = Select(t=w5286, s=w5287, f=w5285) -> (s? t:f=w5284:dbl)
              n3292 = Divide(x=w5291, y=w5284) -> (x/y=w5289:dbl[])
              n3293 = Bundle By Name(cluster=w5290, "magnitude"=w5289) -> (w5288:cluster{"f0":dbl, "df":dbl, "magnitude":dbl[]})
            }
          }
        }
        n3294 = case shown="True" w5230 {
          tunnel: w5231 -> [w5262 w5268]
          tunnel: [w5262 w5263] -> w5229
          frame False {
          }
          frame True {
            n3295 = Array Subset(array=w5268, index (row)=0 ("index"), length (row)=4 ("length"), index (col)=0 ("index"), length (col)=1 ("length")) -> (w5263:T63)
          }
        }
        n3296 = feedback-in #15(w5229) -> ()
        n3297 = Split 1D Array(array=w5243, index=2) -> (first subarray=→"FFT 1":cluster{"f0":dbl, "df":dbl, "magnitude":dbl[]}[], second subarray=→"FFT 2":cluster{"f0":dbl, "df":dbl, "magnitude":dbl[]}[])
      }
    }
    n3298 = local read "Offset Values"() -> (w4319:T20)
    n3299 = local read "T1 calibration"() -> (w4361:T9)
    n3300 = local read "T2 calibration"() -> (w4360:T8)
    n3301 = call-poly <vilib>:"Index Waveform Array.vi"("index"=16, "waveform array"=w4294) -> ("waveform"=w4336:waveform(dbl))  [unwired: 8 in, 1 out]
    n3302 = Unbundle By Name(w4351) -> ("Y"=w4359:dbl[])
    n3303 = Unbundle By Name(w4348) -> ("Y"=w4358:dbl[])
    n3304 = local read "Offset file step size"() -> (w4316:dbl)
    n3305 = Unbundle By Name(w4336) -> ("Y"=→"PSD Y Sum":dbl[])
    n3306 = call "calibrate trap data V2.vi"("Offset File step size"=w4316, "delta frequency"=w4318, "Dynamic offset update"="Dynamic offset\nupdate", "Offsets"=w4319, "T2 cal"=w4360, "T2"=w4358, "T1 cal"=w4361, "T1"=w4359) -> ("T2 force (pN)"=w4352:dbl[], "T2 position (nm)"=w4353:dbl[], "T1 force (pN)"=w4354:dbl[], "T1 position (nm)"=w4355:dbl[])
    n3307 = Bundle By Name(cluster=w4351, "Y"=w4355) -> (w4350:waveform(dbl))
    n3308 = Bundle By Name(cluster=w4351, "Y"=w4354) -> (w4349:waveform(dbl))
    n3309 = Bundle By Name(cluster=w4348, "Y"=w4353) -> (w4347:waveform(dbl))
    n3310 = Bundle By Name(cluster=w4348, "Y"=w4352) -> (w4346:waveform(dbl))
    n3311 = Subtract(x=w4355, y=w4353) -> (x-y=w4516:dbl[])
    n3312 = Negate(x=w4516) -> (-x=w4399:dbl[])
    n3313 = Subtract(x=w4399, y="Offset (nm)") -> (x-y=w4502:dbl[])
    n3314 = case "Choose calibrated display" shown="2" "Calibration" {
      tunnel: w4351 -> [w4931 _ _]
      tunnel: w4348 -> [w4930 _ _]
      tunnel: [w4931 w4933 w4935] -> w4331
      tunnel: [w4930 w4932 w4934] -> w4526
      tunnel: w4350 -> [_ w4933 _]
      tunnel: w4349 -> [_ _ w4935]
      tunnel: w4347 -> [_ w4932 _]
      tunnel: w4346 -> [_ _ w4934]
      frame 0, Default {
      }
      frame 1 {
      }
      frame 2 {
      }
    }
    n3315 = Bundle By Name(cluster=w4351, "Y"=w4502) -> (w4345:waveform(dbl))
    "Bead Separation" <- w4345
    n3316 = feedback #16(w4502) -> (w4501:dbl[])
    n3317 = Build Array (concatenate)(w4502, w4501) -> (w4356:dbl[])
    n3318 = Split 1D Array(array=w4356, index=w4236) -> (first subarray=w4357:dbl[])  [unwired: 1 out]
    n3319 = feedback-in #16(w4357) -> ()
    n3320 = Build Array(w4351, w4350, w4349, w4348, w4347, w4346, w4345) -> (w4344:waveform(dbl)[])
    n3321 = Not(x="Trap Trig. Fl.") -> (.not. x?=w4421:bool)
    n3322 = Unbundle By Name(w4331) -> ("Y"=w4400:dbl[])
    n3323 = Unbundle By Name(w4526) -> ("Y"=w4503:dbl[])
    n3324 = call-poly <vilib>:"Mean.vi"("X"=w4357) -> ("mean"=w4498:dbl)  [unwired: 1 out]
    "Bead Mean (nm)" <- w4498
    n3325 = Multiply(x=w4526, y=-1.0) -> (x*y=w4327:waveform(dbl))
    n3326 = call-poly <vilib>:"Mean.vi"("X"=w4400) -> ("mean"=w4403:dbl)  [unwired: 1 out]
    "T1 X" <- w4403
    n3327 = call-poly <vilib>:"Mean.vi"("X"=w4503) -> ("mean"=w4402:dbl)  [unwired: 1 out]
    "T2 X" <- w4402
    n3328 = Subtract(x=w4357, y=w4498) -> (x-y=w4497:dbl[])
    n3329 = Add(1:w4327, 2:w4331) -> (0:w4330:waveform(dbl))  [unwired: 1 in, 1 out]
    n3330 = Square(x=w4497) -> (x^2=w4496:dbl[])
    n3331 = Divide(x=w4330, y=2.0) -> (x/y=w4328:waveform(dbl))
    n3332 = Negate(x=w4503) -> (-x=w4369:dbl[])
    n3333 = call-poly <vilib>:"Mean.vi"("X"=w4496) -> ("mean"=w4495:dbl)  [unwired: 1 out]
    n3334 = Negate(x=w4402) -> (-x=w4401:dbl)
    n3335 = Square Root(x=w4495) -> (sqrt(x)=w4494:dbl)
    n3336 = Add(x=w4400, y=w4369) -> (x+y=w4504:dbl[])
    n3337 = Add(x=w4403, y=w4401) -> (x+y=w4522:dbl)
    n3338 = Multiply(x=10.0, y=w4494) -> (x*y=→"RMS (Ang)":dbl)
    n3339 = Divide(x=w4504, y=2.0) -> (x/y=w4372:dbl[])
    n3340 = Subtract(x=w4403, y=w4401) -> (x-y=→"Difference":dbl)
    n3341 = Build Array(w4331, w4327, w4328) -> (→"Force":waveform(dbl)[])
    n3342 = Select(t=w4369, s="Only check fixed trap T2", f=w4372) -> (s? t:f=→"Vec Mean of T1 T2":dbl[])
    n3343 = Divide(x=w4522, y=2.0) -> (x/y=w4313:dbl)
    "Mean" <- w4313
    n3344 = feedback-in #17("Trap Trig. Fl.") -> ()
    n3345 = feedback #17("Trap Trig. Fl.") -> (w4419:bool)
    n3346 = And(x=w4421, y=w4419) -> (x .and. y?=w4420:bool)
    n3347 = case "If have just turned off triggering" shown="True" w4420 {
      tunnel: w4324 -> [_ w4748]
      tunnel: w4415 -> [_ w4747]
      frame False {
      }
      frame True {
        w4746 = FALSE ("FPGA Trap Trig")
        n3348 = xnode "Read/Write Control"("FPGA VI Reference In"=w4748, "error in"=w4747, "FPGA Trap Trig"=w4746) -> ("FPGA VI Reference Out"=w4745:T36, "error out"=w4744:errorcluster)
        n3349 = xnode "Read/Write Control"("FPGA VI Reference In"=w4745, "error in"=w4744, "TTrig?"=w4746) -> ()  [unwired: 2 out]
        n3350 = local write "Initializing"(FALSE ("Initializing")) -> ()
        n3351 = local write "Triggered"(FALSE ("Triggered")) -> ()
        n3352 = local write "Waiting"(FALSE ("Waiting")) -> ()
      }
    }
    n3353 = Not(x=w4419) -> (.not. x?=w4432:bool)
    n3354 = And(x="Trap Trig. Fl.", y=w4432) -> (x .and. y?=w4429:bool)
    n3355 = Or(x=w4429, y="Reinitialize") -> (x .or. y?=w4418:bool)
    n3356 = feedback #18(w4425) -> (w4430:string)
    n3357 = Select(t=w4425, s=w4429, f=w4430) -> (s? t:f=w4424:string)
    n3358 = Select(t=w4425, s="Reinitialize", f=w4424) -> (s? t:f=w4423:string)
    n3359 = local read "Tether"() -> (w4506:bool)
    n3360 = feedback #19(0) -> (w4427:i32)
    n3361 = case "For determining if there is a tether still" shown="True" w4506 {
      tunnel: w4313 -> [_ w4857]
      frame False {
      }
      frame True {
        n3362 = Greater?(x="Lost Tether Alarm Threshold (pN)", y=w4857) -> (0:w4855:bool)
        n3363 = case shown="True" w4855 {
          frame False {
          }
          frame True {
            w4858 = FALSE ("Value (Signaling)")
            n3364 = flat-sequence {
              frame #0 {
                # "stop only if saving"
                n3365 = local read "Saving..."() -> (w4870:bool)
                n3366 = And(x=w4870, y="TA Cancel Save?") -> (x .and. y?=w4869:bool)
                n3367 = local write "Stop Saving"(w4869) -> ()
              }
              frame #1 {
                n3368 = case shown="True" "TA Green Off?" {
                  frame False {
                  }
                  frame True {
                    w4873 = FALSE ("Fl. Triggered...")
                    n3369 = local write "Fl. Triggered..."(w4873) -> ()
                    n3370 = property on="Green Laser ON" class="Bool (strict)"("Val(Sgnl)"=w4873) -> ()  [unwired: 2 in, 2 out]
                  }
                }
              }
            }
            n3371 = local read "Time tether formed"() -> (w4864:timestamp)
            n3372 = Get Date/Time In Seconds() -> (seconds since 1Jan1904=w4865:timestamp)
            n3373 = Subtract(x=w4865, y=w4864) -> (x-y=w4863:dbl)
            n3374 = Number To Decimal String(number=w4863) -> (decimal integer string=w4860:string)  [unwired: 1 out]
            n3375 = local read "Messages"() -> (w4867:string)
            n3376 = call <vilib>:"Beep.vi"() -> ()  [unwired: 3 in, 9 out]
            n3377 = Concatenate Strings("Lost tether (" ("Message to add"), w4860, " s)." ("string")) -> (w4862:string)
            n3378 = local write "Tether"(FALSE ("Tether")) -> ()
            n3379 = call "Update messages.vi"("Message to add"=w4862, "Old message string"=w4867) -> ("New message string"=w4866:string)
            n3380 = local write "Messages"(w4866) -> ()
            n3381 = property on="Fl. Triggered..." class="Bool (strict)"("Val(Sgnl)"=w4858) -> ()  [unwired: 2 in, 2 out]
            n3382 = local write "Dip for Protein"(w4858) -> ()
            n3383 = property on="Trap Pos. FB ON" class="Bool (strict)"("Val(Sgnl)"=w4858) -> ()  [unwired: 2 in, 2 out]
            n3384 = property on="Trap Trig. Fl." class="Bool (strict)"("Val(Sgnl)"=w4858) -> ()  [unwired: 2 in, 2 out]
          }
        }
      }
    }
    n3385 = case "For triggering actions based on the trap position (e.g., turning the excitation laser on if trap under feedback moves so far)" shown="True" "Trap Trig. Fl." {
      tunnel: w4229 -> [_ w4761]
      tunnel: w4423 -> [_ w4760]
      tunnel: ["" ("t") w4759] -> w4431
      tunnel: w4418 -> [_ w4758]
      tunnel: [0 ("t") w4757] -> w4428
      tunnel: w4427 -> [_ w4756]
      tunnel: w4324 -> [_ w4755]
      tunnel: w4415 -> [_ w4754]
      frame False {
      }
      frame True {
        n3386 = case shown="\"Wait for trigger\"" w4760 {
          tunnel: w4761 -> [w4778 _ _ w4826]
          tunnel: [w4775 w4807 "" ("t") w4829] -> w4759
          tunnel: w4758 -> [_ _ _ w4817]
          tunnel: [w4774 w4804 0 ("t") w4818] -> w4757
          tunnel: w4756 -> [_ w4806 _ w4824]
          tunnel: w4755 -> [w4763 w4801 _ w4820]
          tunnel: w4754 -> [w4762 w4800 _ w4819]
          frame "Wait for trigger" {
            n3387 = local read "Trap Trig. (FPGA)"() -> (w4766:bool)
            n3388 = Subtract(x=w4778, y="Mean T1 Position\nto compare (nm)") -> (x-y=w4771:dbl[])
            n3389 = call <vilib>:"Std Deviation and Variance.vi"("X"=w4771) -> ("mean"=→"mean":dbl, "standard deviation"=→"standard\ndeviation":dbl)  [unwired: 1 in, 1 out]
            n3390 = Array Max & Min(array=w4771) -> (max value=→"max value":dbl, min value=→"min value":dbl)  [unwired: 2 out]
            n3391 = Greater?(x=w4771, y="Threshold (nm)") -> (0:w4781:bool[])
            n3392 = case shown="True" w4766 {
              tunnel: w4763 -> [_ w4787]
              tunnel: w4762 -> [_ w4786]
              tunnel: [FALSE ("TTrig?") w4785] -> w4769
              frame False {
              }
              frame True {
                n3393 = xnode "Read/Write Control"("FPGA VI Reference In"=w4787, "error in"=w4786) -> ("TTrig?"=w4785:bool)  [unwired: 2 out]
              }
            }
            n3394 = Or Array Elements(Boolean array=w4781) -> (logical OR=w4768:bool)
            n3395 = Select(t=w4769, s=w4766, f=w4768) -> (s? t:f=w4767:bool)
            n3396 = Not(x=w4766) -> (.not. x?=w4765:bool)
            n3397 = And(x=w4767, y=w4765) -> (x .and. y?=w4764:bool)
            n3398 = Select(t="Triggered", s=w4767, f="Wait for trigger") -> (s? t:f=w4775:string)
            n3399 = case shown="True" w4767 {
              tunnel: [0 0] -> w4774
              tunnel: w4763 -> [_ w4792]
              tunnel: w4762 -> [_ w4791]
              frame False {
                "Waiting" <- TRUE ("Waiting")
              }
              frame True {
                n3400 = xnode "Read/Write Control"("FPGA VI Reference In"=w4792, "error in"=w4791, "TTrig?"=FALSE) -> ()  [unwired: 2 out]
                n3401 = local read "Messages"() -> (w4795:string)
                n3402 = call <vilib>:"Beep.vi"() -> ()  [unwired: 12 in]
                n3403 = call "Update messages.vi"("Message to add"="Unwinding trigger.", "Old message string"=w4795) -> ("New message string"=w4796:string)
                n3404 = local write "Messages"(w4796) -> ()
                n3405 = local write "Waiting"(FALSE ("Waiting")) -> ()
                "Triggered" <- TRUE ("Triggered")
              }
            }
            n3406 = case "Only need to turn on laser if host triggered" shown="True" w4764 {
              frame False {
              }
              frame True {
                n3407 = property on="Green Laser ON" class="Bool (strict)"("Val(Sgnl)"=TRUE ("Value (Signaling)")) -> ()  [unwired: 2 in, 2 out]
              }
            }
          }
          frame "Triggered" {
            n3408 = local read "Trap Trig. (FPGA)"() -> (w4803:bool)
            n3409 = Increment(x=w4806) -> (x+1=w4804:i32)
            n3410 = Greater Or Equal?(x=w4804, y="Fl. ON time (n)") -> (x >= y?=w4802:bool)
            n3411 = Select(t="Wait for trigger", s=w4802, f="Triggered" ("t")) -> (s? t:f=w4807:string)
            n3412 = And(x=w4802, y=w4803) -> (x .and. y?=w4799:bool)
            n3413 = case shown="True" w4799 {
              tunnel: w4801 -> [_ w4811]
              tunnel: w4800 -> [_ w4810]
              frame False {
              }
              frame True {
                n3414 = xnode "Read/Write Control"("FPGA VI Reference In"=w4811, "error in"=w4810, "FPGA Trap Trig"=TRUE) -> ()  [unwired: 2 out]
              }
            }
            n3415 = case shown="True" w4802 {
              frame False {
              }
              frame True {
                w4813 = FALSE ("Value (Signaling)")
                n3416 = local write "Triggered"(w4813) -> ()
                n3417 = local write "Waiting"(TRUE ("Waiting")) -> ()
                n3418 = property on="Green Laser ON" class="Bool (strict)"("Val(Sgnl)"=w4813) -> ()  [unwired: 2 in, 2 out]
              }
            }
          }
          frame "Do nothing" {
          }
          frame "Initialize", Default {
            n3419 = Increment(x=w4824) -> (x+1=w4828:i32)
            n3420 = Select(t=1, s=w4817, f=w4828) -> (s? t:f=w4818:i32)
            n3421 = feedback #20(w4826) -> (w4832:dbl[])
            n3422 = Build Array (concatenate)(w4826, w4832) -> (w4825:dbl[])
            n3423 = Greater Or Equal?(x=w4818, y="Wait to get offset (n)") -> (x >= y?=w4821:bool)
            n3424 = Select(t=w4826, s=w4817, f=w4825) -> (s? t:f=w4827:dbl[])
            n3425 = feedback-in #20(w4827) -> ()
            n3426 = call-poly <vilib>:"Mean.vi"("X"=w4827) -> ("mean"=w4822:dbl)  [unwired: 1 out]
            n3427 = local write "Mean T1 Position\nto compare (nm)"(w4822) -> ()
            n3428 = case shown="True" w4817 {
              tunnel: w4820 -> [_ w4838]
              tunnel: w4819 -> [_ w4837]
              frame False {
              }
              frame True {
                w4834 = FALSE ("FPGA Trap Trig")
                n3429 = xnode "Read/Write Control"("FPGA VI Reference In"=w4838, "error in"=w4837, "FPGA Trap Trig"=w4834) -> ("FPGA VI Reference Out"=w4836:T36, "error out"=w4835:errorcluster)
                n3430 = xnode "Read/Write Control"("FPGA VI Reference In"=w4836, "error in"=w4835, "TTrig?"=w4834) -> ()  [unwired: 2 out]
              }
            }
            n3431 = Select(t="Wait for trigger", s=w4821, f="Initialize") -> (s? t:f=w4829:string)
            n3432 = case shown="True" w4821 {
              tunnel: w4822 -> [_ w4841]
              tunnel: w4820 -> [_ w4850]
              tunnel: w4819 -> [_ w4849]
              frame False {
                n3433 = local write "Waiting"(FALSE ("Waiting")) -> ()
                "Initializing" <- TRUE ("Initializing")
              }
              frame True {
                n3434 = local read "Threshold (nm)"() -> (w4853:dbl)
                n3435 = local read "AOM X Cal (nm/MHz)"() -> (w4852:dbl)
                n3436 = Add(x=w4841, y=w4853) -> (x+y=w4854:dbl)
                n3437 = Divide(x=w4854, y=w4852) -> (x/y=w4851:dbl)
                n3438 = call "IR AOM freq to word.vi"("Frequency In (MHz)"=w4851) -> ("Frequency Word Out (double)"=w4848:dbl)
                n3439 = local write "Initializing"(FALSE ("Initializing")) -> ()
                n3440 = local write "Waiting"(TRUE ("Waiting")) -> ()
                n3441 = To Quad Integer(1:w4848) -> (0:w4847:i64)
                n3442 = xnode "Read/Write Control"("FPGA VI Reference In"=w4850, "error in"=w4849, "FPGA TTrig Thresh"=w4847) -> ("FPGA VI Reference Out"=w4844:T36, "error out"=w4843:errorcluster)
                n3443 = xnode "Read/Write Control"("FPGA VI Reference In"=w4844, "error in"=w4843, "FPGA Trap Trig"=TRUE) -> ()  [unwired: 2 out]
              }
            }
          }
        }
      }
    }
    n3444 = feedback-in #18(w4431) -> ()
    n3445 = feedback-in #19(w4428) -> ()
    n3446 = xnode ("Read/Write Control")("FPGA VI Reference In"=w4223, "error in"=w4514) -> ("FPGA VI Reference Out"=w4315:T36, "error out"=w4416:errorcluster, "AI2 Y Sum Set 1"=w4563:i16, "AI2 Y Sum Set 2"=w4562:i16, "AI1 X Set 1"=w4454:fxp<+/-,16,1>, "AI1 X Set 2"=w4453:fxp<+/-,16,1>, "Trap Pos FB Int Signal"=→"Trap Pos FB Int Signal":fxp<+/-,24,9>, "Trap Pos FB Int-Norm Signal"=→"Trap Pos FB Int-Norm Signal":fxp<+/-,16,1>, "Trap Pos FB Action"=w4447:i64, "Scanning"=→"AOD Scanning":bool, "Scan I"=→"AOD Scan I":u64, "Scanning MCL"=w4565:bool, "Scan I (MCL)"=→"MCL Scan I":u64, "Green FB Sum"=w4527:i16, "Trap Pos FB Action"=w4414:i64, "TTrig Fin Thresh"=w4410:i64, "Red FB Intensity"=w4397:i16, "Blue Intensity"=w4392:i16, "BD1 Frequency Out 1"=w4332:u64)
    "MCL Scanning" <- w4565
    "Trap Pos FB Action" <- w4447
    n3447 = Divide(x=w4397, y=3276.7) -> (x/y=w4396:dbl)
    "Red laser intensity (V)" <- w4396
    n3448 = Divide(x=w4392, y=3276.7) -> (x/y=w4391:dbl)
    "Blue laser intensity (V)" <- w4391
    n3449 = Divide(x=w4527, y=3276.7) -> (x/y=w4395:dbl)
    "Green laser intensity (V)" <- w4395
    n3450 = local read "FB Trig Integrate"() -> (w4408:u32)
    n3451 = Divide(x=w4414, y=w4408) -> (x/y=w4407:dbl)
    "TTrig Sig (Int)" <- w4407
    n3452 = Bundle(w4395, w4396, w4391) -> (→"Fluorescence laser intensities plot":cluster{dbl, dbl, dbl})  [unwired: 1 in]
    n3453 = Divide(x=w4410, y=w4408) -> (x/y=w4405:dbl)
    "TTrig Fin Thresh (Int)" <- w4405
    n3454 = local read "AOM X Cal (nm/MHz)"() -> (w4413:dbl)
    n3455 = local read "AI2 (V)"() -> (w4564:cluster{"Set 1":dbl, "Set 2":dbl})
